vi "Teleop.vi"(10 "Match Info":T2={"Autonomous Elapsed Seconds"=0.0, "TeleOp Elapsed Seconds"=0.0, "Disabled Elapsed Seconds"=0.0, "Visited Autonomous"=FALSE, "Visited TeleOp"=FALSE, "Visited Disabled"=FALSE, "Autonomous Settings"={"Autonomous Style"=enum."Independent", "VI Refnum"=refnum}}, 11 "Call Context":T3) -> ()   [LabVIEW 2012]
doc: "This VI is called for each TeleOp packet received from the DS where the robot is not disabled. It is often used to read from the joysticks and update I/O or to update setpoints for timed control loops. It should complete and return within 20 milliseconds or it may miss DS packets."
uses:
  <vilib>/Rock Robotics/WPI/DriverStation/WPI_DriverStationDerivedRobotMode.ctl
  <vilib>/Rock Robotics/WPI/DriverStation/WPI_DriverStationMatch Info.ctl
  <vilib>/Rock Robotics/WPI/Relay/WPI_RelayValue.ctl
  Robot Global Data.vi
  <vilib>/Rock Robotics/WPI/Joystick/WPI_JoystickGetSetRefNum.vi
panel:
  in  "Harvestor":T1
  in  "Indexer":dbl
  in  "Rollers":dbl
  in  "FlipperUp":bool
  in  "Flipper2Up":dbl=110.0
  in  "Flipper2Down":dbl=110.0
  in  "Flipper1Down":dbl=110.0
  in  "Flipper1Up":dbl=110.0
  in  "ShooterWheelB":dbl
  in  "ShooterWheelF":dbl
  in  "Dep Const":dbl=0.5
  in  "Roller Speed":dbl=0.75
  in  "RelayValue 2":T1
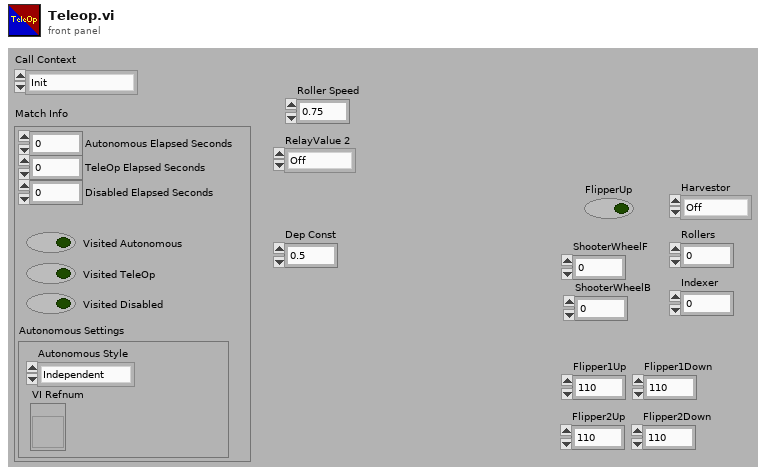
[diagram p1: front panel]
types:
  T1 = typedef "WPI_RelayValue.ctl" = enum16{"Off", "On", "Forward", "Reverse"}
  T2 = typedef "WPI_DriverStationMatch Info.ctl" = cluster{"Autonomous Elapsed Seconds":dbl, "TeleOp Elapsed Seconds":dbl, "Disabled Elapsed Seconds":dbl, "Visited Autonomous":bool, "Visited TeleOp":bool, "Visited Disabled":bool, "Autonomous Settings":cluster{"Autonomous Style":enum16{"Iterative", "Independent"}, "VI Refnum":refnum<vi>}}
  T3 = typedef "WPI_DriverStationDerivedRobotMode.ctl" = enum16{"Init", "Execute", "Stop"}
  T4 = typedef "WPI_ServoDeviceRef.ctl" = cluster{"DeviceStatus":errorcluster, "Digital Module":T5, "PWM Channel":T6, "DeadBand":T7}
  T5 = typedef "FPGA_TypedefDigitalModule.ctl" = enum16{"Digital Module 1", "Digital Module 2"}
  T6 = typedef "FPGA_DIOPWMChannel.ctl" = enum8{"PWM 1", "PWM 2", "PWM 3", "PWM 4", "PWM 5", "PWM 6", "PWM 7", "PWM 8", "PWM 9", "PWM 10", "Invalid"}
  T7 = typedef "WPI_PWMDeadband.ctl" = cluster{"Name":string, "maxPositivePwm":i32, "minPositivePwm":i32, "centerPwm":i32, "maxNegativePwm":i32, "minNegativePwm":i32, "angularRange":u16}
  T8 = typedef "WPI_MotorControlDeviceRef.ctl" = cluster{"DeviceStatus":errorcluster, "Type":enum16{"PWM", "CAN"}, "PWM":cluster{"Digital Module":T5, "PWM Channel":T6, "DeadBand":T7}, "CAN":cluster{"Device Number":u8, "Control Mode":T9, "Semaphore":T10, "Max Vout":dbl}, "Invert":bool, "TransformRef":T11, "InvTransformRef":T11}
  T9 = typedef "WPI_CANJaguar_ControlMode.ctl" = enum8{"Percent VBus", "Current", "Speed", "Position", "Voltage"}
  T10 = typedef "Semaphore RefNum" = refnum<k1>
  T11 = typedef "WPI_PWMTransform_ConPane.ctl" = refnum<vi>
  T12 = typedef "WPI_RelayDevRef.ctl" = cluster{"DevStatus":errorcluster, "Relay Channel":T13, "Digital Module":T5, "Relay Direction":T14}
  T13 = typedef "FPGA_DIORelayChannel.ctl" = enum8{"Relay 1", "Relay 2", "Relay 3", "Relay 4", "Relay 5", "Relay 6", "Relay 7", "Relay 8", "Invalid"}
  T14 = typedef "WPI_RelayDirection.ctl" = enum16{"Both directions", "Forward only", "Reverse only"}
  T15 = cluster{"Driver Station Digital Input (1-8)[0]":bool, "Driver Station Digital Input (1-8)[1]":bool, "Driver Station Digital Input (1-8)[2]":bool, "Driver Station Digital Input (1-8)[3]":bool, "Driver Station Digital Input (1-8)[4]":bool, "Driver Station Digital Input (1-8)[5]":bool, "Driver Station Digital Input (1-8)[6]":bool, "Driver Station Digital Input (1-8)[7]":bool, "Driver Station Digital Input (1-8)[8]":bool}
  T16 = cluster{"Right Servo High":dbl, "Right Servo Mid":dbl, "Right Servo Low":dbl, "Left Servo High":dbl, "Left Servo Mid":dbl, "Left Servo Low":dbl}
  T17 = typedef "WPI_JoystickDevRef.ctl" = cluster{"Device":T18}
  T18 = typedef "WPI_JoystickDeviceEnum.ctl" = enum16{"USB 1", "USB 2", "USB 3", "USB 4", "Kinect 1", "Kinect 2"}
  T19 = cluster{"axis 1 (x)":dbl, "axis 2 (y)":dbl, "axis 3 (throttle)":dbl, "axis 4":dbl, "axis 5":dbl, "axis 6":dbl}
  T20 = typedef "WPI_JoystickButtonState.ctl" = cluster{"Button 1":bool, "Button 2":bool, "Button 3":bool, "Button 4":bool, "Button 5":bool, "Button 6":bool, "Button 7":bool, "Button 8":bool, "Button 9":bool, "Button 10":bool, "Button 11":bool, "Button 12":bool}
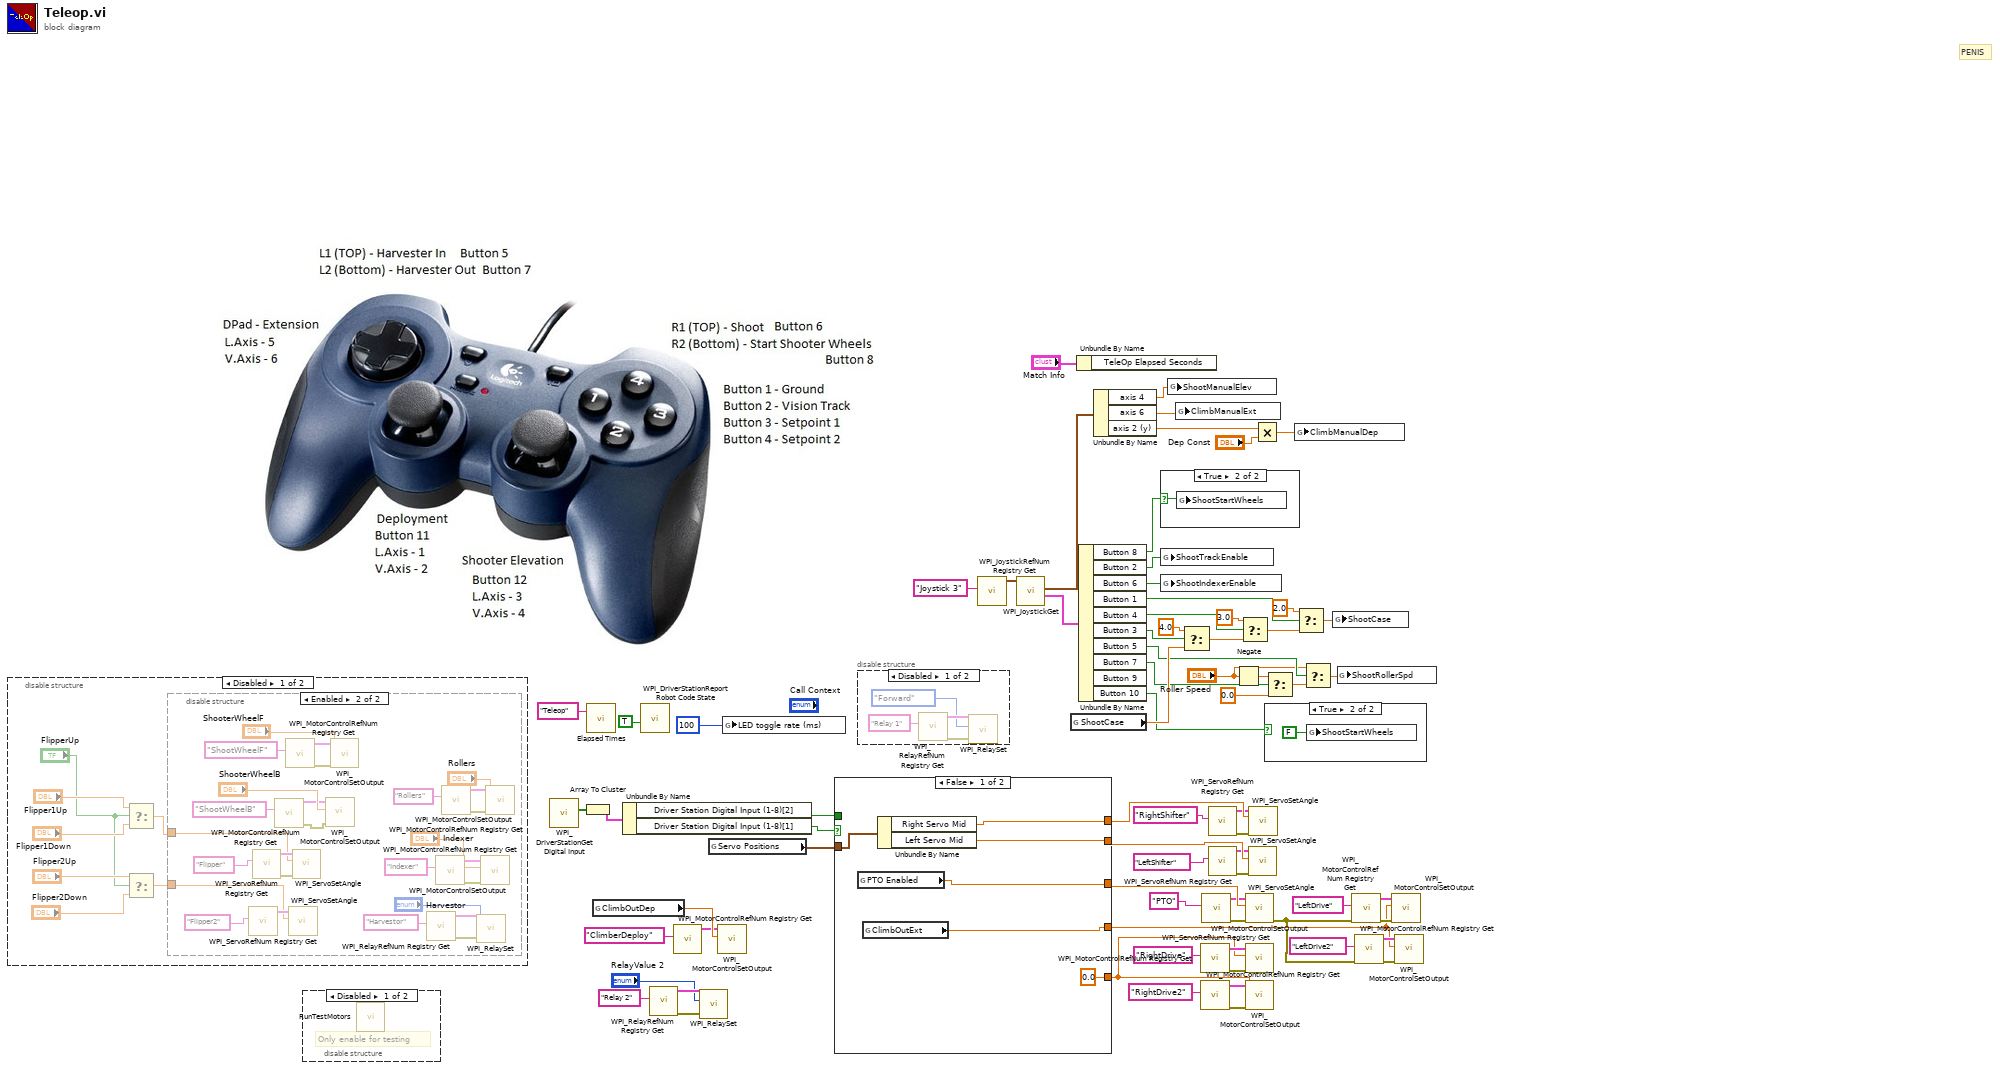
[diagram p0: block diagram]
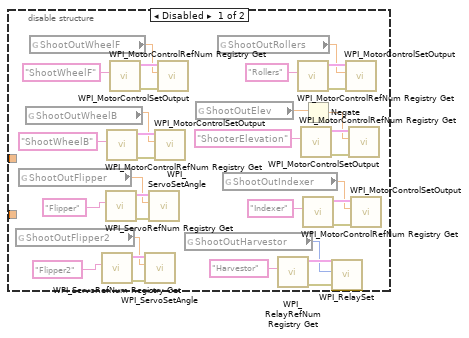
[diagram p4: hidden frame]
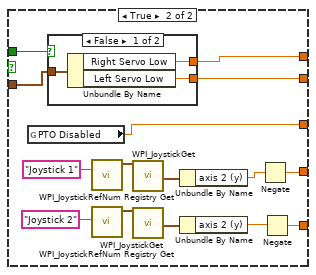
[diagram p6: hidden frame]
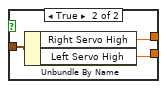
[diagram p7: hidden frame]
diagram:
  # "PENIS"
  n1 = disable-structure shown="Disabled" {
    frame Disabled {
      n2 = Select(t="Flipper1Up", s="FlipperUp", f="Flipper1Down") -> (s? t:f=w75:dbl)
      n3 = Select(t="Flipper2Up", s="FlipperUp", f="Flipper2Down") -> (s? t:f=w74:dbl)
      n4 = disable-structure shown="Enabled" {
        disable-tunnel: w75 -> [_ w127]
        disable-tunnel: w74 -> [_ w126]
        frame Disabled {
          n5 = global read "Robot Global Data.vi" "ShootOutFlipper2"() -> (w85:dbl)
          n6 = global read "Robot Global Data.vi" "ShootOutFlipper"() -> (w86:dbl)
          n7 = global read "Robot Global Data.vi" "ShootOutWheelB"() -> (w93:dbl)
          n8 = global read "Robot Global Data.vi" "ShootOutWheelF"() -> (w98:dbl)
          n9 = call <vilib>:"WPI_ServoRefNum Registry Get.vi"("refnum name"="Flipper2") -> ("error out"=w89:errorcluster, "ServoDeviceRef"=w88:T4)  [unwired: 9 in]
          n10 = call <vilib>:"WPI_ServoRefNum Registry Get.vi"("refnum name"="Flipper") -> ("error out"=w90:errorcluster, "ServoDeviceRef"=w91:T4)  [unwired: 9 in]
          n11 = call <vilib>:"WPI_MotorControlRefNum Registry Get.vi"("refnum name"="ShootWheelB") -> ("error out"=w108:errorcluster, "MotorControlDevRef"=w109:T8)  [unwired: 9 in]
          n12 = call <vilib>:"WPI_MotorControlRefNum Registry Get.vi"("refnum name"="ShootWheelF") -> ("error out"=w113:errorcluster, "MotorControlDevRef"=w112:T8)  [unwired: 9 in]
          n13 = call <vilib>:"WPI_ServoSetAngle.vi"("error in (no error)"=w89, "Angle"=w85, "ServoDeviceRef"=w88) -> ()  [unwired: 7 in, 2 out]
          n14 = call <vilib>:"WPI_ServoSetAngle.vi"("error in (no error)"=w90, "Angle"=w86, "ServoDeviceRef"=w91) -> ()  [unwired: 7 in, 2 out]
          n15 = call <vilib>:"WPI_MotorControlSetOutput.vi"("error in (no error)"=w108, "Output"=w93, "MotorControlDevRef"=w109) -> ()  [unwired: 6 in, 3 out]
          n16 = call <vilib>:"WPI_MotorControlSetOutput.vi"("error in (no error)"=w113, "Output"=w98, "MotorControlDevRef"=w112) -> ()  [unwired: 6 in, 3 out]
          n17 = global read "Robot Global Data.vi" "ShootOutHarvestor"() -> (w81:T1)
          n18 = global read "Robot Global Data.vi" "ShootOutElev"() -> (w95:dbl)
          n19 = global read "Robot Global Data.vi" "ShootOutRollers"() -> (w96:dbl)
          n20 = global read "Robot Global Data.vi" "ShootOutIndexer"() -> (w97:dbl)
          n21 = call <vilib>:"WPI_RelayRefNum Registry Get.vi"("refnum name"="Harvestor") -> ("error out"=w84:errorcluster, "RelayDevRef"=w82:T12)  [unwired: 9 in]
          n22 = call <vilib>:"WPI_MotorControlRefNum Registry Get.vi"("refnum name"="Rollers") -> ("error out"=w105:errorcluster, "MotorControlDevRef"=w106:T8)  [unwired: 9 in]
          n23 = call <vilib>:"WPI_MotorControlRefNum Registry Get.vi"("refnum name"="ShooterElevation") -> ("error out"=w104:errorcluster, "MotorControlDevRef"=w103:T8)  [unwired: 9 in]
          n24 = Negate(x=w95) -> (-x=w94:dbl)
          n25 = call <vilib>:"WPI_MotorControlRefNum Registry Get.vi"("refnum name"="Indexer") -> ("error out"=w99:errorcluster, "MotorControlDevRef"=w100:T8)  [unwired: 9 in]
          n26 = call <vilib>:"WPI_RelaySet.vi"("error in (no error)"=w84, "RelayValue"=w81, "RelayDevRef"=w82) -> ()  [unwired: 7 in, 2 out]
          n27 = call <vilib>:"WPI_MotorControlSetOutput.vi"("error in (no error)"=w105, "Output"=w96, "MotorControlDevRef"=w106) -> ()  [unwired: 6 in, 3 out]
          n28 = call <vilib>:"WPI_MotorControlSetOutput.vi"("error in (no error)"=w104, "Output"=w94, "MotorControlDevRef"=w103) -> ()  [unwired: 6 in, 3 out]
          n29 = call <vilib>:"WPI_MotorControlSetOutput.vi"("error in (no error)"=w99, "Output"=w97, "MotorControlDevRef"=w100) -> ()  [unwired: 6 in, 3 out]
        }
        frame Enabled {
          n30 = call <vilib>:"WPI_ServoRefNum Registry Get.vi"("refnum name"="Flipper2") -> ("ServoDeviceRef"=w137:T4)  [unwired: 9 in, 1 out]
          n31 = call <vilib>:"WPI_ServoRefNum Registry Get.vi"("refnum name"="Flipper") -> ("error out"=w136:errorcluster, "ServoDeviceRef"=w135:T4)  [unwired: 9 in]
          n32 = call <vilib>:"WPI_MotorControlRefNum Registry Get.vi"("refnum name"="ShootWheelB") -> ("error out"=w119:errorcluster, "MotorControlDevRef"=w120:T8)  [unwired: 9 in]
          n33 = call <vilib>:"WPI_MotorControlRefNum Registry Get.vi"("refnum name"="ShootWheelF") -> ("error out"=w115:errorcluster, "MotorControlDevRef"=w116:T8)  [unwired: 9 in]
          n34 = call <vilib>:"WPI_ServoSetAngle.vi"("Angle"=w126, "ServoDeviceRef"=w137) -> ()  [unwired: 8 in, 2 out]
          n35 = call <vilib>:"WPI_ServoSetAngle.vi"("error in (no error)"=w136, "Angle"=w127, "ServoDeviceRef"=w135) -> ()  [unwired: 7 in, 2 out]
          n36 = call <vilib>:"WPI_MotorControlSetOutput.vi"("error in (no error)"=w119, "Output"="ShooterWheelB", "MotorControlDevRef"=w120) -> ()  [unwired: 6 in, 3 out]
          n37 = call <vilib>:"WPI_MotorControlSetOutput.vi"("error in (no error)"=w115, "Output"="ShooterWheelF", "MotorControlDevRef"=w116) -> ()  [unwired: 6 in, 3 out]
          n38 = call <vilib>:"WPI_RelayRefNum Registry Get.vi"("refnum name"="Harvestor") -> ("error out"=w123:errorcluster, "RelayDevRef"=w140:T12)  [unwired: 9 in]
          n39 = call <vilib>:"WPI_MotorControlRefNum Registry Get.vi"("refnum name"="Indexer") -> ("error out"=w133:errorcluster, "MotorControlDevRef"=w132:T8)  [unwired: 9 in]
          n40 = call <vilib>:"WPI_MotorControlRefNum Registry Get.vi"("refnum name"="Rollers") -> ("error out"=w130:errorcluster, "MotorControlDevRef"=w129:T8)  [unwired: 9 in]
          n41 = call <vilib>:"WPI_RelaySet.vi"("error in (no error)"=w123, "RelayValue"="Harvestor", "RelayDevRef"=w140) -> ()  [unwired: 7 in, 2 out]
          n42 = call <vilib>:"WPI_MotorControlSetOutput.vi"("error in (no error)"=w133, "Output"="Indexer", "MotorControlDevRef"=w132) -> ()  [unwired: 6 in, 3 out]
          n43 = call <vilib>:"WPI_MotorControlSetOutput.vi"("error in (no error)"=w130, "Output"="Rollers", "MotorControlDevRef"=w129) -> ()  [unwired: 6 in, 3 out]
        }
      }
    }
    frame Enabled {
    }
  }
  n44 = disable-structure shown="Disabled" {
    frame Disabled {
      # "Only enable for testing"
      n45 = call "RunTestMotors.vi"() -> ()  [unwired: 16 in]
    }
    frame Enabled {
    }
  }
  n46 = call <vilib>:"WPI_DriverStationGet Digital Input.vi"() -> ("Driver Station Digital Input (1-8)"=w33:bool[])  [unwired: 11 in]
  n47 = Array To Cluster(array=w33) -> (cluster=w32:T15)
  n48 = call "Elapsed Times.vi"("Call Name"="Teleop") -> ()  [unwired: 2 in, 1 out]
  n49 = global read "Robot Global Data.vi" "ClimbOutDep"() -> (w17:dbl)
  n50 = Unbundle By Name(w32) -> ("Driver Station Digital Input (1-8)[2]"=w31:bool, "Driver Station Digital Input (1-8)[1]"=w23:bool)
  n51 = call <vilib>:"WPI_DriverStationReport Robot Code State.vi"("TeleOp"=TRUE ("Autonomous")) -> ()  [unwired: 10 in, 1 out]
  n52 = call <vilib>:"WPI_RelayRefNum Registry Get.vi"("refnum name"="Relay 2") -> ("error out"=w2:errorcluster, "RelayDevRef"=w4:T12)  [unwired: 9 in]
  n53 = call <vilib>:"WPI_MotorControlRefNum Registry Get.vi"("refnum name"="ClimberDeploy") -> ("MotorControlDevRef"=w15:T8)  [unwired: 9 in, 1 out]
  n54 = call <vilib>:"WPI_RelaySet.vi"("error in (no error)"=w2, "RelayValue"="RelayValue 2", "RelayDevRef"=w4) -> ()  [unwired: 7 in, 2 out]
  n55 = global read "Robot Global Data.vi" "Servo Positions"() -> (w30:T16)
  n56 = call <vilib>:"WPI_MotorControlSetOutput.vi"("Output"=w17, "MotorControlDevRef"=w15) -> ()  [unwired: 7 in, 3 out]
  n57 = global write "Robot Global Data.vi" "LED toggle rate (ms)"(u32 100 ("LED ms toggle rate")) -> ()
  n58 = case shown="False" w23 {
    tunnel: w31 -> [_ w161]
    tunnel: w30 -> [w146 w160]
    tunnel: [w145 w159] -> w29
    tunnel: [w144 w158] -> w28
    tunnel: [w143 w157] -> w20
    tunnel: [w141 w148] -> w19
    tunnel: [0.0 w147] -> w18
    frame False {
      n59 = global read "Robot Global Data.vi" "PTO Enabled"() -> (w143:dbl)
      n60 = global read "Robot Global Data.vi" "ClimbOutExt"() -> (w141:dbl)
      n61 = Unbundle By Name(w146) -> ("Right Servo Mid"=w145:dbl, "Left Servo Mid"=w144:dbl)
    }
    frame True {
      n62 = global read "Robot Global Data.vi" "PTO Disabled"() -> (w157:dbl)
      n63 = case shown="False" w161 {
        tunnel: w160 -> [w164 w167]
        tunnel: [w163 w166] -> w159
        tunnel: [w162 w165] -> w158
        frame False {
          n64 = Unbundle By Name(w164) -> ("Right Servo Low"=w163:dbl, "Left Servo Low"=w162:dbl)
        }
        frame True {
          n65 = Unbundle By Name(w167) -> ("Right Servo High"=w166:dbl, "Left Servo High"=w165:dbl)
        }
      }
      n66 = call <vilib>:"WPI_JoystickRefNum Registry Get.vi"("refnum name"="Joystick 1") -> ("JoystickDevRef"=w149:T17)  [unwired: 1 in, 9 out]
      n67 = call <vilib>:"WPI_JoystickRefNum Registry Get.vi"("refnum name"="Joystick 2") -> ("JoystickDevRef"=w155:T17)  [unwired: 1 in, 9 out]
      n68 = call <vilib>:"WPI_JoystickGet.vi"("JoystickDevRef"=w149) -> ("Axes"=w152:T19)  [unwired: 1 in, 5 out]
      n69 = call <vilib>:"WPI_JoystickGet.vi"("JoystickDevRef"=w155) -> ("Axes"=w156:T19)  [unwired: 1 in, 5 out]
      n70 = Unbundle By Name(w152) -> ("axis 2 (y)"=w151:dbl)
      n71 = Unbundle By Name(w156) -> ("axis 2 (y)"=w153:dbl)
      n72 = Negate(x=w151) -> (-x=w148:dbl)
      n73 = Negate(x=w153) -> (-x=w147:dbl)
    }
  }
  n74 = disable-structure shown="Disabled" {
    frame Disabled {
      n75 = call <vilib>:"WPI_RelayRefNum Registry Get.vi"("refnum name"="Relay 1") -> ("error out"=w169:errorcluster, "RelayDevRef"=w171:T12)  [unwired: 9 in]
      n76 = call <vilib>:"WPI_RelaySet.vi"("error in (no error)"=w169, "RelayValue"=WPI_RelayValue."Forward", "RelayDevRef"=w171) -> ()  [unwired: 7 in, 2 out]
    }
    frame Enabled {
    }
  }
  n77 = call <vilib>:"WPI_JoystickRefNum Registry Get.vi"("refnum name"="Joystick 3") -> ("JoystickDevRef"=w70:T17)  [unwired: 9 in, 1 out]
  n78 = call <vilib>:"WPI_JoystickGet.vi"("JoystickDevRef"=w70) -> ("Buttons"=w68:T20, "Axes"=w67:T19)  [unwired: 4 in, 1 out]
  n79 = global read "Robot Global Data.vi" "ShootCase"() -> (w55:dbl)
  n80 = Unbundle By Name("Match Info") -> ()  [unwired: 1 out]
  n81 = Unbundle By Name(w68) -> ("Button 8"=w48:bool, "Button 2"=w65:bool, "Button 6"=w66:bool, "Button 1"=w63:bool, "Button 4"=w61:bool, "Button 3"=w60:bool, "Button 5"=w51:bool, "Button 7"=w53:bool, "Button 10"=w47:bool)  [unwired: 1 out]
  n82 = Unbundle By Name(w67) -> ("axis 4"=w64:dbl, "axis 6"=w1:dbl, "axis 2 (y)"=w7:dbl)
  n83 = case shown="True" w48 {
    selector: w48 -> [_ w172]
    frame False {
    }
    frame True {
      n84 = global write "Robot Global Data.vi" "ShootStartWheels"(w172) -> ()
    }
  }
  n85 = global write "Robot Global Data.vi" "ShootTrackEnable"(w65) -> ()
  n86 = global write "Robot Global Data.vi" "ShootIndexerEnable"(w66) -> ()
  n87 = global write "Robot Global Data.vi" "ShootManualElev"(w64) -> ()
  n88 = global write "Robot Global Data.vi" "ClimbManualExt"(w1) -> ()
  n89 = Select(t=4.0, s=w60, f=w55) -> (s? t:f=w59:dbl)
  n90 = call <vilib>:"WPI_MotorControlRefNum Registry Get.vi"("refnum name"="RightDrive") -> ("error out"=w43:errorcluster, "MotorControlDevRef"=w45:T8)  [unwired: 9 in]
  n91 = call <vilib>:"WPI_MotorControlRefNum Registry Get.vi"("refnum name"="RightDrive2") -> ("error out"=w36:errorcluster, "MotorControlDevRef"=w34:T8)  [unwired: 9 in]
  n92 = call <vilib>:"WPI_ServoRefNum Registry Get.vi"("refnum name"="PTO") -> ("error out"=w13:errorcluster, "ServoDeviceRef"=w14:T4)  [unwired: 9 in]
  n93 = call <vilib>:"WPI_ServoRefNum Registry Get.vi"("refnum name"="RightShifter") -> ("error out"=w24:errorcluster, "ServoDeviceRef"=w25:T4)  [unwired: 9 in]
  n94 = call <vilib>:"WPI_ServoRefNum Registry Get.vi"("refnum name"="LeftShifter") -> ("error out"=w26:errorcluster, "ServoDeviceRef"=w27:T4)  [unwired: 9 in]
  n95 = Negate(x="Roller Speed") -> (-x=w11:dbl)
  n96 = Select(t=3.0, s=w61, f=w59) -> (s? t:f=w57:dbl)
  n97 = call <vilib>:"WPI_ServoSetAngle.vi"("error in (no error)"=w13, "Angle"=w20, "ServoDeviceRef"=w14) -> ("error out"=w6:errorcluster)  [unwired: 7 in, 1 out]
  n98 = call <vilib>:"WPI_MotorControlSetOutput.vi"("error in (no error)"=w43, "Output"=w18, "MotorControlDevRef"=w45) -> ()  [unwired: 6 in, 3 out]
  n99 = call <vilib>:"WPI_MotorControlSetOutput.vi"("error in (no error)"=w36, "Output"=w18, "MotorControlDevRef"=w34) -> ()  [unwired: 6 in, 3 out]
  n100 = call <vilib>:"WPI_ServoSetAngle.vi"("error in (no error)"=w26, "Angle"=w28, "ServoDeviceRef"=w27) -> ()  [unwired: 7 in, 2 out]
  n101 = call <vilib>:"WPI_ServoSetAngle.vi"("error in (no error)"=w24, "Angle"=w29, "ServoDeviceRef"=w25) -> ()  [unwired: 7 in, 2 out]
  n102 = Multiply(x=w7, y="Dep Const") -> (x*y=w9:dbl)
  n103 = case shown="True" w47 {
    frame False {
    }
    frame True {
      n104 = global write "Robot Global Data.vi" "ShootStartWheels"(FALSE ("ShootStartWheels")) -> ()
    }
  }
  n105 = Select(t=w11, s=w53, f=0.0) -> (s? t:f=w52:dbl)
  n106 = global write "Robot Global Data.vi" "ClimbManualDep"(w9) -> ()
  n107 = Select(t=2.0, s=w63, f=w57) -> (s? t:f=w54:dbl)
  n108 = Select(t="Roller Speed", s=w51, f=w52) -> (s? t:f=w49:dbl)
  n109 = global write "Robot Global Data.vi" "ShootCase"(w54) -> ()
  n110 = global write "Robot Global Data.vi" "ShootRollerSpd"(w49) -> ()
  n111 = call <vilib>:"WPI_MotorControlRefNum Registry Get.vi"("error in (no error)"=w6, "refnum name"="LeftDrive") -> ("error out"=w38:errorcluster, "MotorControlDevRef"=w41:T8)  [unwired: 8 in]
  n112 = call <vilib>:"WPI_MotorControlRefNum Registry Get.vi"("error in (no error)"=w6, "refnum name"="LeftDrive2") -> ("error out"=w37:errorcluster, "MotorControlDevRef"=w39:T8)  [unwired: 8 in]
  n113 = call <vilib>:"WPI_MotorControlSetOutput.vi"("error in (no error)"=w38, "Output"=w19, "MotorControlDevRef"=w41) -> ()  [unwired: 6 in, 3 out]
  n114 = call <vilib>:"WPI_MotorControlSetOutput.vi"("error in (no error)"=w37, "Output"=w19, "MotorControlDevRef"=w39) -> ()  [unwired: 6 in, 3 out]
